vi "uActor_Disable AutoACK.vi"(8 "error in (no error)":errorcluster, 11 "uActor in":refnum<class "uActor.lvclass">) -> (0 "error out":errorcluster, 3 "uActor out":refnum<class "uActor.lvclass">)   [LabVIEW 2023, in "uLib.lvlib" / "uActor.lvclass"]
doc: "Call this method to prevent the actor from sending auto ack messages or auto reply meesages as it processes the incoming commands.\n<B>Disabling auto replies will result in ignoring any replies wired to the output terminal of the EXEC method.</B>\n\nThis is relevant for message dispatching actors that should not send out an Ack or a reply on their own but leave that to the destination actor. It is also relevant for observer actors that should passively monitor (and/or log) events but should not actively engage in replying to senders."
uses:
  uActor.lvclass
  uActor.lvclass/uActor.ctl
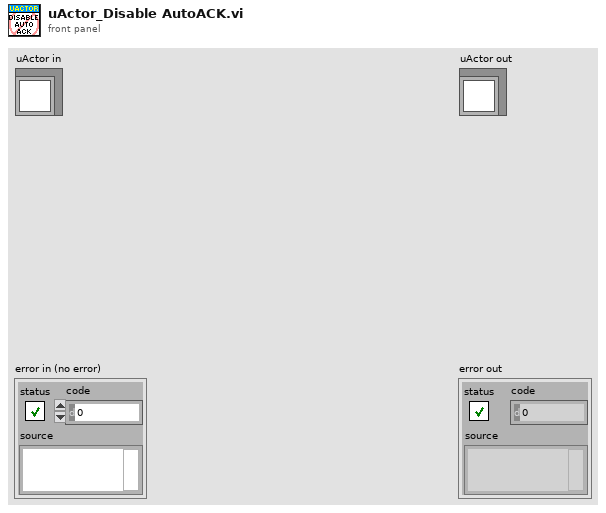
[diagram p1: front panel]
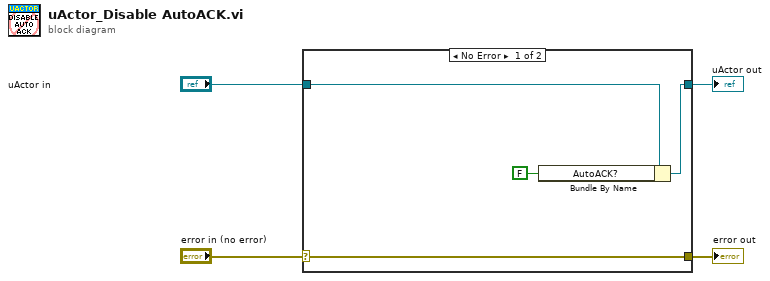
[diagram p0: block diagram]
diagram:
  n1 = case shown="No Error" "error in (no error)" {
    selector: "error in (no error)" -> [w8 w9]
    tunnel: [w8 w9] -> w3
    tunnel: [w6 w10] -> w1
    tunnel: "uActor in" -> [w7 w10]
    frame No Error {
      n2 = Bundle By Name(cluster=w7, "AutoACK?"=FALSE ("RnT config.AutoACK?")) -> (w6:refnum<class "uActor.lvclass">)
    }
    frame Error {
    }
  }
  "error out" <- w3
  "uActor out" <- w1
